vi "High_Sample_Waveforms.vi"(8 "millisecond multiple":u32) -> (1 "L3 Current":waveform(dbl)[](graph), 2 "L2 Current":waveform(dbl)[](graph), 3 "L1 Current":waveform(dbl)[](graph), 9 "L3 Voltage":waveform(dbl)[](graph), 10 "L2 Voltage":waveform(dbl)[](graph), 11 "L1 Voltage":waveform(dbl)[](graph))   [LabVIEW 2019]
uses:
  <vilib>/DAQmx/read.llb/DAQmx Read (Analog 1D Wfm NChan NSamp).vi
  <vilib>/DAQmx/miscellaneous.llb/DAQmx Fill In Error Info.vi
  <vilib>/Waveform/WDTOps.llb/WDT Index Channel DBL.vi
panel:
  out "error out":errorcluster
  in  "error in":errorcluster
  out "Waveform Graph":waveform(dbl)[](graph)
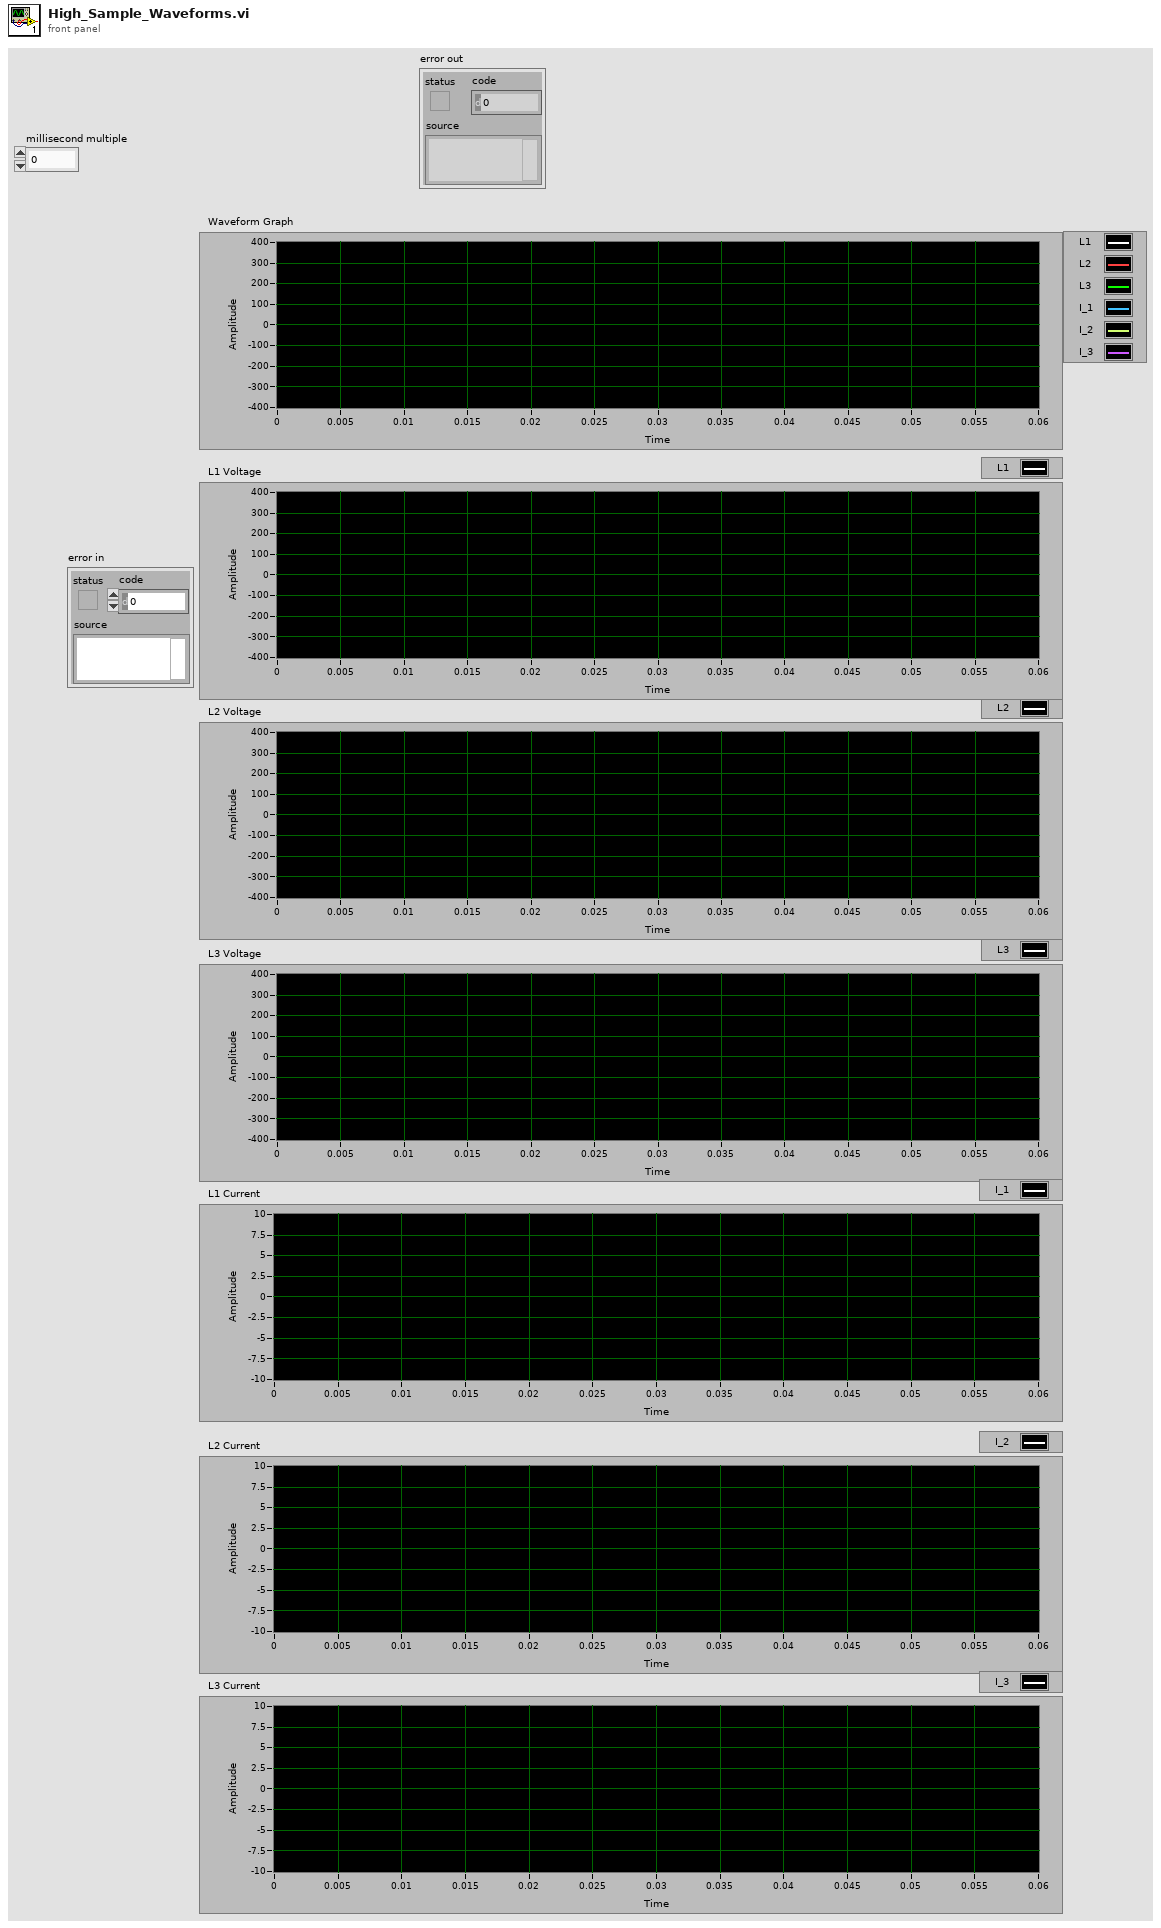
[diagram p1: front panel]
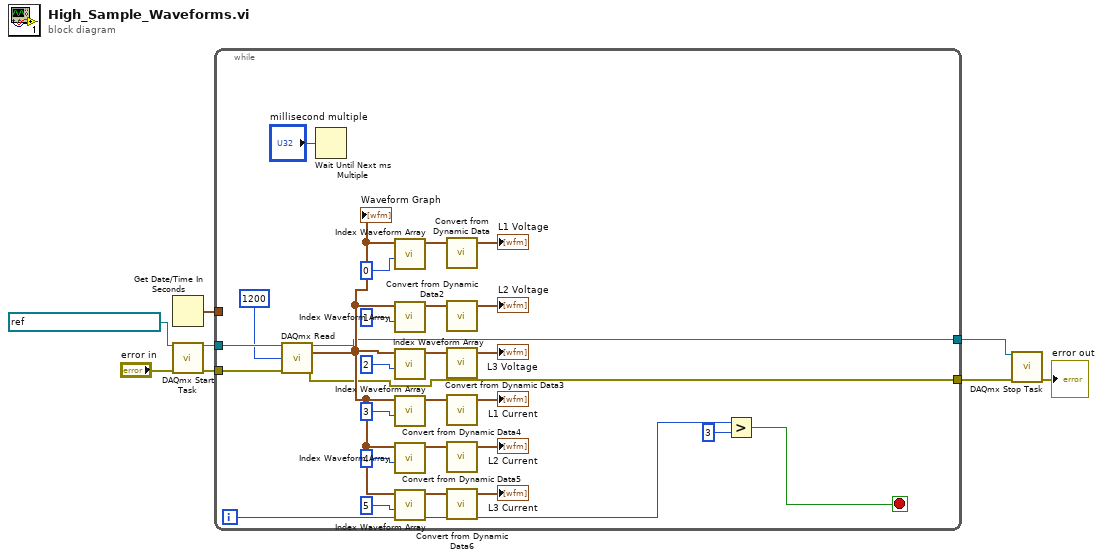
[diagram p0: block diagram]
diagram:
  n1 = Get Date/Time In Seconds() -> (seconds since 1Jan1904=w4:timestamp)
  n2 = call <vilib>:"DAQmx Start Task.vi"("task/channels in"=refnum<k21> "PTS_CAB1kHighSample", "error in"="error in") -> ("task out"=w6:refnum<k21>, "error out"=w5:errorcluster)  [unwired: 12 in]
  n3 = while {
    tunnel: w6 -> [w36]
    tunnel: w5 -> [w35]
    tunnel: w4 -> [_]
    tunnel: [w10] -> w3
    tunnel: [w9] -> w2
    i -> [w14]
    stop <- w12 stop-if-true
    n4 = call-poly <vilib>:"DAQmx Read.vi"("task/channels in"=w36, "number of samples per channel"=1200, "error in"=w35) -> ("task out"=w9:refnum<k21>, "data"=w17:waveform(dbl)[], "error out"=w10:errorcluster)  [unwired: 10 in]
    "Waveform Graph" <- w17
    n5 = Wait Until Next ms Multiple(millisecond multiple="millisecond multiple") -> ()  [unwired: 1 out]
    n6 = call-poly <vilib>:"Index Waveform Array.vi"("index"=0, "waveform array"=w17) -> ("waveform"=w11:waveform(dbl))  [unwired: 8 in, 1 out]
    n7 = call-poly <vilib>:"Index Waveform Array.vi"("index"=1, "waveform array"=w17) -> ("waveform"=w23:waveform(dbl))  [unwired: 8 in, 1 out]
    n8 = call-poly <vilib>:"Index Waveform Array.vi"("index"=2, "waveform array"=w17) -> ("waveform"=w24:waveform(dbl))  [unwired: 8 in, 1 out]
    n9 = call-poly <vilib>:"Index Waveform Array.vi"("index"=3, "waveform array"=w17) -> ("waveform"=w25:waveform(dbl))  [unwired: 8 in, 1 out]
    n10 = call-poly <vilib>:"Index Waveform Array.vi"("index"=4, "waveform array"=w17) -> ("waveform"=w26:waveform(dbl))  [unwired: 8 in, 1 out]
    n11 = call-poly <vilib>:"Index Waveform Array.vi"("index"=5, "waveform array"=w17) -> ("waveform"=w28:waveform(dbl))  [unwired: 8 in, 1 out]
    n12 = call "Convert from Dynamic Data"("Dynamic Data Type"=w11) -> ("Array of Waveform"=→"L1 Voltage":waveform(dbl)[])  [unwired: 3 in]
    n13 = call "Convert from Dynamic Data2"("Dynamic Data Type"=w23) -> ("Array of Waveform"=→"L2 Voltage":waveform(dbl)[])  [unwired: 3 in]
    n14 = call "Convert from Dynamic Data3"("Dynamic Data Type"=w24) -> ("Array of Waveform"=→"L3 Voltage":waveform(dbl)[])  [unwired: 3 in]
    n15 = call "Convert from Dynamic Data4"("Dynamic Data Type"=w25) -> ("Array of Waveform"=→"L1 Current":waveform(dbl)[])  [unwired: 3 in]
    n16 = call "Convert from Dynamic Data5"("Dynamic Data Type"=w26) -> ("Array of Waveform"=→"L2 Current":waveform(dbl)[])  [unwired: 3 in]
    n17 = call "Convert from Dynamic Data6"("Dynamic Data Type"=w28) -> ("Array of Waveform"=→"L3 Current":waveform(dbl)[])  [unwired: 3 in]
    n18 = Greater?(x=w14, y=3) -> (0:w12:bool)
  }
  n19 = call <vilib>:"DAQmx Stop Task.vi"("task/channels in"=w2, "error in"=w3) -> ("error out"=→"error out":errorcluster)  [unwired: 12 in, 1 out]
